vi "Pre Launch Init.vi"(11 "LS-H600-TCP Client in":refnum<class "LS-H600-TCP Client.lvclass"> caption="操作者输入") -> (0 "error out":errorcluster caption="错误输出", 3 "LS-H600-TCP Client out":refnum<class "LS-H600-TCP Client.lvclass"> caption="操作者输出")   [LabVIEW 2016, in "LS-H600-TCP Client.lvlib" / "LS-H600-TCP Client.lvclass"]
doc: "(<B>Filename</B>: Actor Framework.lvlib:Actor.lvclass:Pre Launch Init.vi)\n\nDefines behavior that occurs after the Launch Nested Actor method is invoked but before the actor's Actor Core method begins running.\n\nBy default, this method does nothing.子孙类重写该方法定义具体的操作。"
uses:
  LS-H600-TCP Client.lvclass
  <vilib>/ActorFramework/Actor/Actor.lvclass
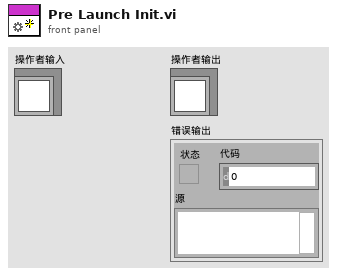
[diagram p1: front panel]
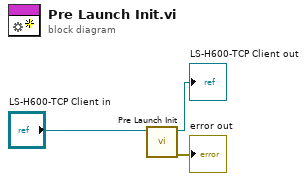
[diagram p0: block diagram]
diagram:
  n1 = call-parent "Pre Launch Init.vi"("Actor in"="LS-H600-TCP Client in") -> ("error out"=→"error out":errorcluster, "Actor out"=→"LS-H600-TCP Client out":refnum<class "LS-H600-TCP Client.lvclass">)  [unwired: 9 in]
